vi "虚拟家庭血压仪.vi"() -> ()   [LabVIEW 2016]
uses:
  <vilib>/Analysis/2dsp.llb/Real FFT.vi
  <vilib>/Analysis/NI_AALPro.lvlib
  <vilib>/Analysis/NI_AAL_SigProc.lvlib
  <vilib>/measure/NI_MABase.lvlib
panel:
  in  "?":bool
  out "?":string[][](table)
  in  "?":i32(ring) items=["0", "1", "2", "3", "4", "5", "6", "7", "8", "9", "10", "11", "12", "13", "14", "15", "16", "17", "18", "19", "20"]
  in  "电源":bool
  out "本月血压波形":cluster{"初始x轴值":i32, "△X":i32, i64[][]}(graph)
  in  "?":bool
  in  "?":bool
  in  "?":bool
  out "采集窗口":dynamicdata(graph)
  out "舒张压":i32
  out "收缩压":i32
  out "?":bool
  out "?":string
  out "?":string
  out "?":bool
  out "心率":i32
  out "?":bool
  out "?":string
  out "?":string
  # "虚   拟  家  庭   血   压   仪"
  # "显  示  面  板"
  # "家庭成员信息录入"
  # "成员选择"
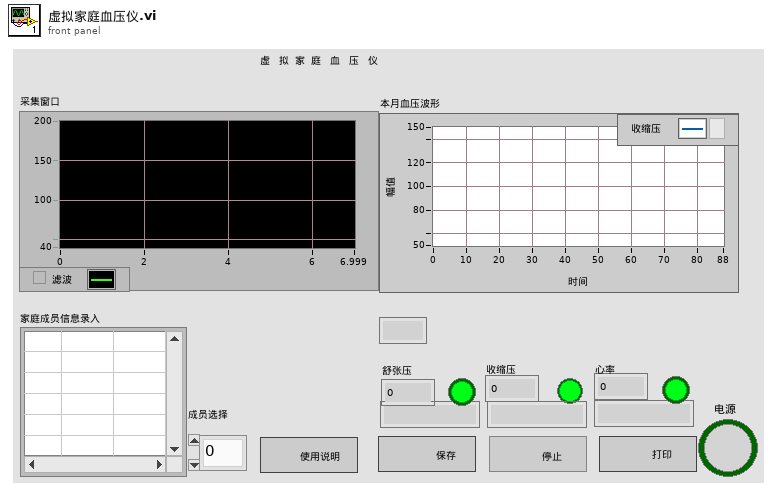
[diagram p1: front panel]
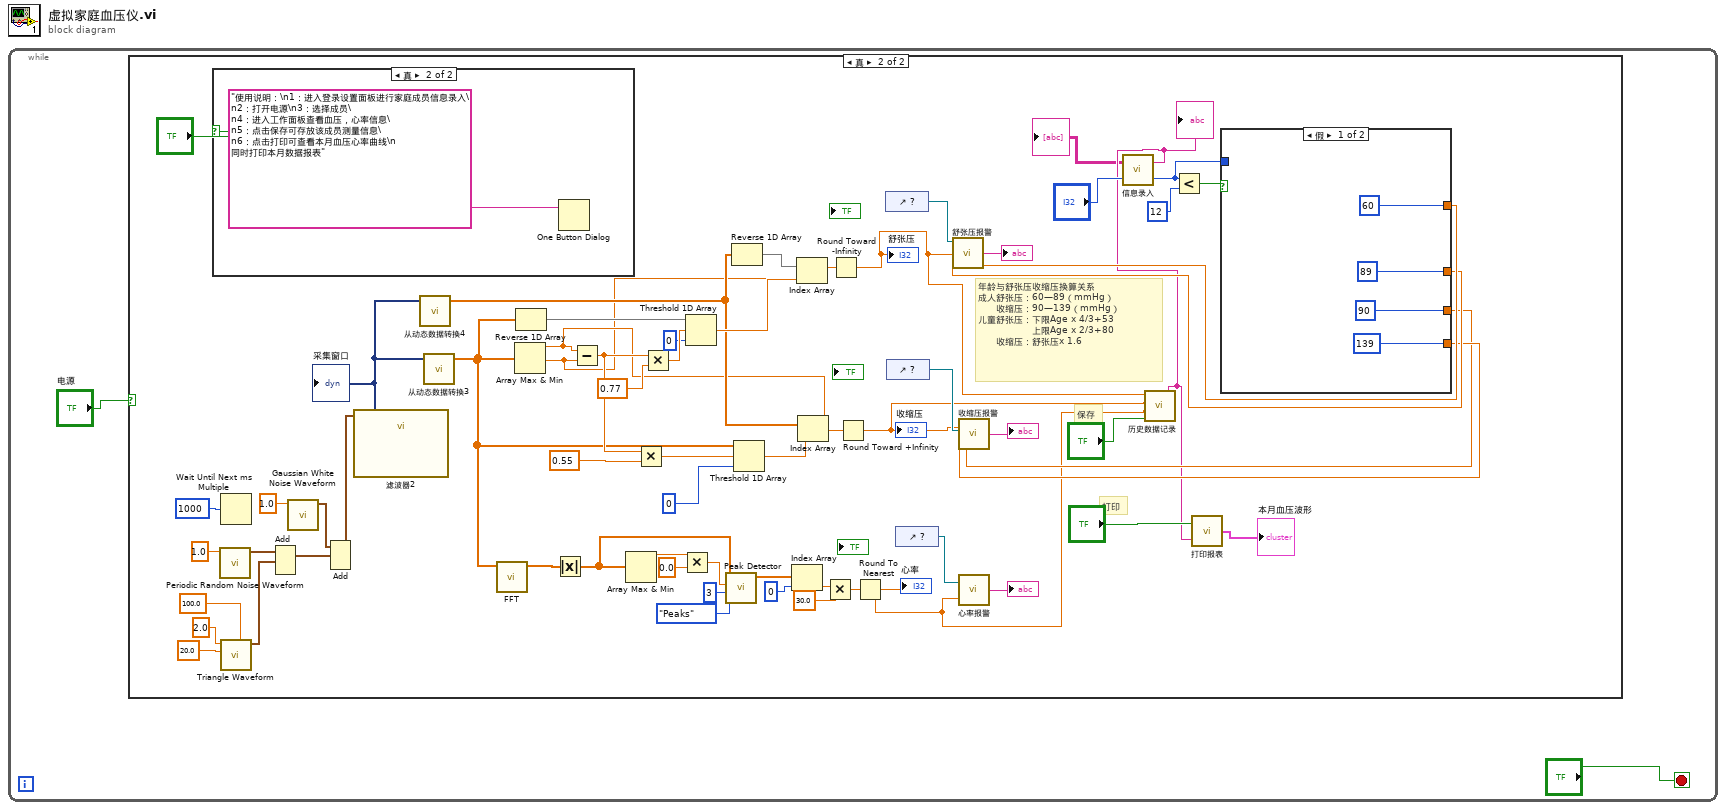
[diagram p0: block diagram]
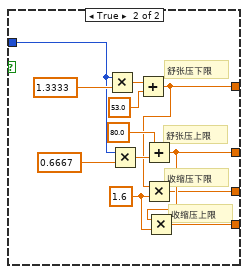
[diagram p4: hidden frame]
diagram:
  n1 = while {
    stop <- "?" stop-if-true
    n2 = case shown="真" "电源" {
      frame False {
      }
      frame True {
        # "打印"
        # "保存"
        # "年龄与舒张压收缩压换算关系\n成人舒张压：60—89（mmHg）\n      收缩压：90—139（mmHg）\n儿童舒张压：下限Age x 4/3+53\n                  上限Age x 2/3+80 \n      收缩压：舒张压x 1.6"
        n3 = case shown="真" "?" {
          frame False {
          }
          frame True {
            n4 = One Button Dialog(message="使用说明：\n1：进入登录设置面板进行家庭成员信息录入\n2：打开电源\n3：选择成员\n4：进入工作面板查看血压，心率信息\n5：点击保存可存放该成员测量信息\n6：点击打印可查看本月血压心率曲线\n     同时打印本月数据报表" ("消息")) -> ()  [unwired: 1 in, 1 out]
          }
        }
        n5 = call <vilib>:"Periodic Random Noise Waveform.vi"("spectral amplitude"=1.0 ("mean")) -> ("signal out"=w13:waveform(dbl))  [unwired: 9 in, 1 out]
        n6 = Wait Until Next ms Multiple(millisecond multiple=u32 1000 ("毫秒倍数")) -> ()  [unwired: 1 out]
        n7 = call <vilib>:"Triangle Waveform.vi"("offset"=100.0, "amplitude"=20.0, "frequency"=2.0) -> ("signal out"=w17:waveform(dbl))  [unwired: 7 in, 1 out]
        n8 = Add(1:w17, 2:w13) -> (0:w16:waveform(dbl))  [unwired: 1 in, 1 out]
        n9 = call <vilib>:"Gaussian White Noise Waveform.vi"("standard deviation"=1.0 ("amplitude")) -> ("signal out"=w20:waveform(dbl))  [unwired: 9 in, 1 out]
        n10 = Add(1:w16, 2:w20) -> (0:w12:waveform(dbl))  [unwired: 1 in, 1 out]
        n11 = call "滤波器2"("Signal"=w12) -> ("Filtered Signal"=w37:dynamicdata)  [unwired: 9 in, 1 out]
        "采集窗口" <- w37
        n12 = call "从动态数据转换4"("Dynamic Data Type"=w37) -> ("Array"=w53:dbl[])  [unwired: 3 in]
        n13 = call "从动态数据转换3"("Dynamic Data Type"=w37) -> ("Array"=w48:dbl[])  [unwired: 3 in]
        n14 = call-poly <vilib>:"FFT.vi"("X"=w48) -> ("FFT {X}"=w47:cdb[])  [unwired: 9 in, 1 out]
        n15 = Array Max & Min(array=w48) -> (max value=w4:dbl, min value=w3:dbl)  [unwired: 2 out]
        n16 = Reverse 1D Array(array=w48) -> (reversed array=w64:dbl[])
        n17 = Absolute Value(x=w47) -> (abs(x)=w43:dbl[])
        n18 = Subtract(x=w4, y=w3) -> (x-y=w62:dbl)
        n19 = Array Max & Min(array=w43) -> (max value=w46:dbl)  [unwired: 3 out]
        n20 = Multiply(x=w62, y=0.55) -> (x*y=w59:dbl)
        n21 = Multiply(x=w62, y=0.77) -> (x*y=w57:dbl)
        n22 = Multiply(x=w46, y=0.0) -> (x*y=w44:dbl)
        n23 = Threshold 1D Array(1:0 ("开始索引(0)"), 2:w57, 3:w64) -> (0:w54:dbl)
        n24 = call <vilib>:"Peak Detector.vi"("peaks/valleys"=enum32{"Peaks", "Valleys"}."Peaks", "width"=3, "threshold"=w44, "X"=w43) -> ("Locations"=w41:dbl[])  [unwired: 3 in, 4 out]
        n25 = Reverse 1D Array(array=w53) -> (reversed array=w55:dbl[])
        n26 = Threshold 1D Array(1:0 ("开始索引(0)"), 2:w59, 3:w48) -> (0:w58:dbl)
        n27 = Index Array(array=w41, index=0 ("索引")) -> (element=w8:dbl)
        n28 = Index Array(array=w55, index=w54) -> ()  [unwired: 1 out]
        n29 = Index Array(array=w53, index=w58) -> ()  [unwired: 1 out]
        n30 = Multiply(x=w8, y=30.0) -> (x*y=w6:dbl)
        n31 = Round Toward -Infinity(1:w3) -> (0:w11:dbl)
        "舒张压" <- w11
        n32 = Round Toward +Infinity(x=w4) -> (ceil(x): smallest int >= x=w10:dbl)
        "收缩压" <- w10
        n33 = Round To Nearest(number=w6) -> (nearest integer value=w5:dbl)
        "心率" <- w5
        n34 = control-ref of="?"() -> (w52:refnum<vi>)
        n35 = control-ref of="?"() -> (w49:refnum<vi>)
        n36 = control-ref of="?"() -> (w39:refnum<vi>)
        n37 = call "心率报警.vi"(1:"心率"=w5, 2:"心率"=w39) -> ("心率情况"=→"?":string)
        n38 = call "信息录入.vi"(2:"?") -> ("年龄 2"=w33:u8, "成员 2"=w26:string, "表格控件"=→"?":string[][])
        "?" <- w26
        n39 = call "历史数据记录.vi"("成员信息"=w26, 1:"?", "心率"=w5, "收缩压"=w10, "舒张压"=w11) -> ()
        n40 = Less?(x=w33, y=u8 12) -> (x < y?=w34:bool)
        n41 = call "打印报表.vi"("成员信息"=w26, 2:"?") -> (0:→"本月血压波形":cluster{"初始x轴值":i32, "△X":i32, i64[][]})
        n42 = case shown="假" w34 {
          tunnel: w33 -> [_ w77]
          tunnel: [60 w73] -> w32
          tunnel: [89 w72] -> w31
          tunnel: [90 w71] -> w29
          tunnel: [139 w70] -> w30
          frame False {
          }
          frame True {
            w74 = 1.6 ("y")
            # "收缩压上限"
            # "收缩压下限"
            # "舒张压上限"
            # "舒张压下限"
            n43 = Multiply(x=w77, y=1.3333) -> (x*y=w80:dbl)
            n44 = Multiply(x=w77, y=0.6667) -> (x*y=w76:dbl)
            n45 = Add(x=w80, y=53.0) -> (x+y=w73:dbl)
            n46 = Add(x=80.0, y=w76) -> (x+y=w72:dbl)
            n47 = Multiply(x=w73, y=w74) -> (x*y=w71:dbl)
            n48 = Multiply(x=w72, y=w74) -> (x*y=w70:dbl)
          }
        }
        n49 = call "舒张压报警.vi"("舒张压下限"=w32, "舒张压上限"=w31, "舒张压"=w11, "警示 2"=w52) -> ("预警 2"=→"?":string)
        n50 = call "收缩压报警.vi"("收缩压下限"=w29, "收缩压上限"=w30, 3:"收缩压"=w49, 4:"收缩压"=w10) -> ("收缩压情况"=→"?":string)
      }
    }
  }
